vi "ReadCICDPathConfig.vi"(8 "error in (no error)":errorcluster, 11 "Workspace Path":path=path "E:/sw-deps-monitor") -> (0 "error out":errorcluster, 3 "CICD Path Config Out":T1)   [LabVIEW 2023, in "CICD.lvlib"]
uses:
  CICD.lvlib
  Typedefs/CICDPathConfigs.ctl
  <vilib>/Utility/config.llb/NI_LVConfig.lvlib
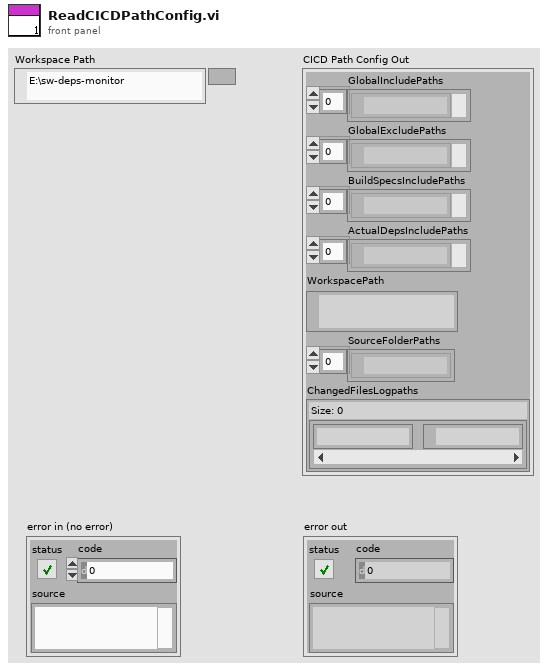
[diagram p1: front panel]
types:
  T1 = typedef "CICD.lvlib/CICDPathConfigs.ctl" = cluster{"GlobalIncludePaths":path[], "GlobalExcludePaths":path[], "BuildSpecsIncludePaths":path[], "ActualDepsIncludePaths":path[], "WorkspacePath":path, "SourceFolderPaths":path[], "ChangedFilesLogpaths":map{string, path}}
  T2 = typedef "NI_LVConfig.lvlib/Config Data RefNum.ctl" = refnum<k1>
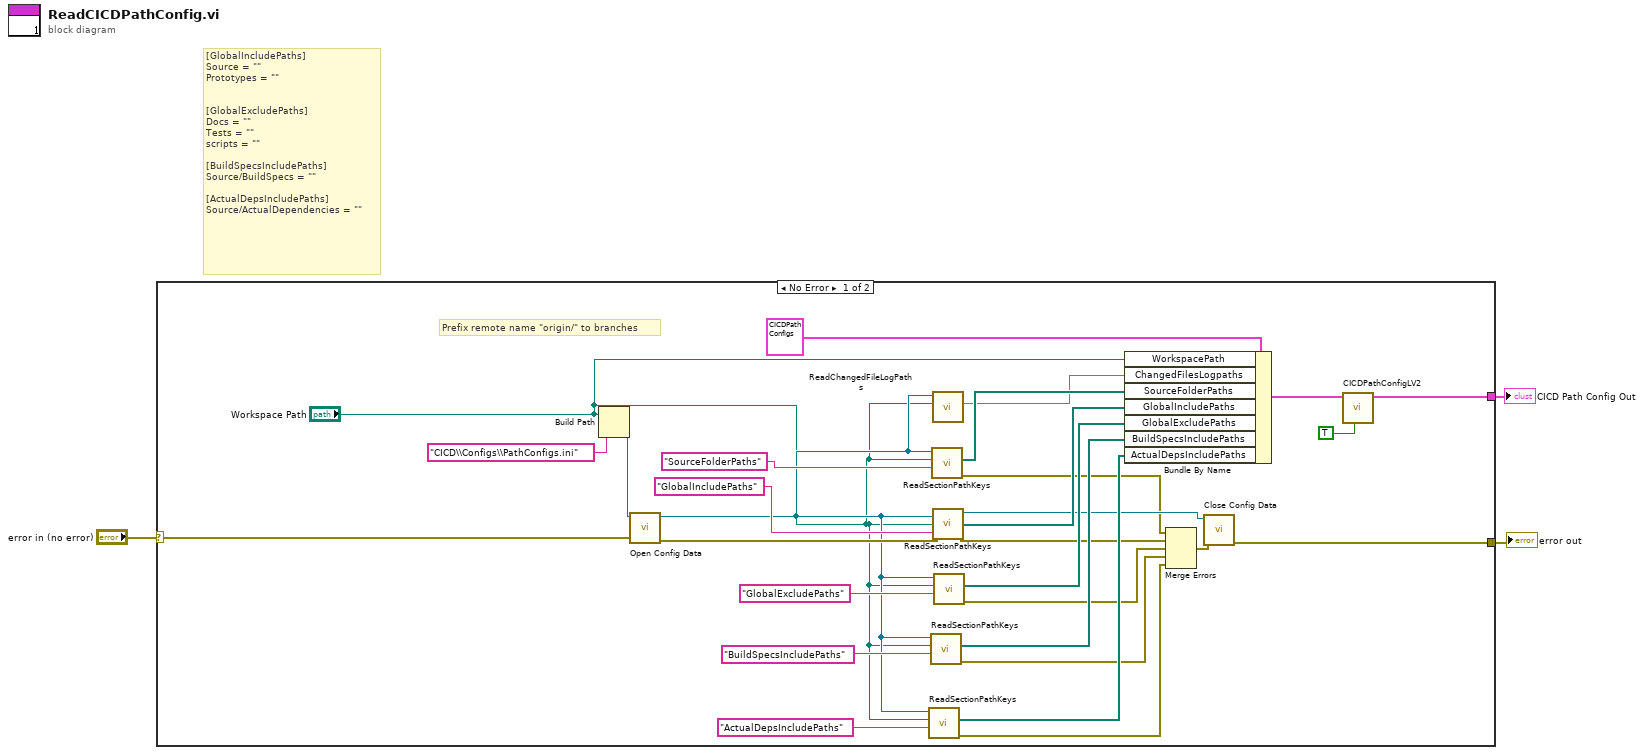
[diagram p0: block diagram]
diagram:
  # "[GlobalIncludePaths]\nSource = \"\"\nPrototypes = \"\"\n\n\n[GlobalExcludePaths]\nDocs = \"\"\nTests = \"\"\nscripts = \"\"\n\n[BuildSpecsIncludePaths]\nSource/BuildSpecs = \"\"\n\n[ActualDepsIncludePaths]\nSource/ActualDependencies = \"\""
  n1 = case shown="No Error" "error in (no error)" {
    selector: "error in (no error)" -> [w32 w33]
    tunnel: [w13 w33] -> w2
    tunnel: [w10 _] -> w1
    frame No Error {
      # "Prefix remote name \"origin/\" to branches"
      n2 = Build Path(base path="Workspace Path", name or relative path="CICD\\Configs\\PathConfigs.ini" ("CICD Path Config Rel")) -> (appended path=w31:path)
      n3 = call <vilib>:"Open Config Data.vi"("error in (no error)"=w32, "configuration file path"=w31) -> ("error out"=w29:errorcluster, "refnum"=w6:T2)  [unwired: 7 in, 1 out]
      n4 = call "ReadSectionPathKeys.vi"("section"="ActualDepsIncludePaths", "Workspace Path"="Workspace Path", "Refnum in"=w6) -> ("error out"=w16:errorcluster, "Paths"=w20:path[])  [unwired: 6 in, 1 out]
      n5 = call "ReadSectionPathKeys.vi"("section"="BuildSpecsIncludePaths", "Workspace Path"="Workspace Path", "Refnum in"=w6) -> ("error out"=w17:errorcluster, "Paths"=w21:path[])  [unwired: 6 in, 1 out]
      n6 = call "ReadSectionPathKeys.vi"("section"="SourceFolderPaths", "Workspace Path"="Workspace Path", "Refnum in"=w6) -> ("error out"=w8:errorcluster, "Paths"=w7:path[])  [unwired: 6 in, 1 out]
      n7 = call "ReadChangedFileLogPaths.vi"("Workspace Path"="Workspace Path", "Refnum in"=w6) -> ("ChangedFilesLogpaths"=w4:map{string, path})  [unwired: 7 in, 2 out]
      n8 = call "ReadSectionPathKeys.vi"("error in (no error)"=w29, "section"="GlobalIncludePaths", "Workspace Path"="Workspace Path", "Refnum in"=w6) -> ("error out"=w19:errorcluster, "Paths"=w23:path[], "refnum out"=w14:T2)  [unwired: 5 in]
      n9 = call "ReadSectionPathKeys.vi"("section"="GlobalExcludePaths", "Workspace Path"="Workspace Path", "Refnum in"=w6) -> ("error out"=w18:errorcluster, "Paths"=w22:path[])  [unwired: 6 in, 1 out]
      n10 = Bundle By Name(cluster=T1 {"GlobalIncludePaths"=[], "GlobalExcludePaths"=[], "BuildSpecsIncludePaths"=[], "ActualDepsIncludePaths"=[], "WorkspacePath"=path "", "SourceFolderPaths"=[], "ChangedFilesLogpaths"={}}, "WorkspacePath"="Workspace Path", "ChangedFilesLogpaths"=w4, "SourceFolderPaths"=w7, "GlobalIncludePaths"=w23, "GlobalExcludePaths"=w22, "BuildSpecsIncludePaths"=w21, "ActualDepsIncludePaths"=w20) -> (w11:T1)
      n11 = Merge Errors(w8, w19, w18, w17, w16) -> (w15:errorcluster)
      n12 = call <vilib>:"Close Config Data.vi"("error in (no error)"=w15, "refnum"=w14) -> ("error out"=w13:errorcluster)  [unwired: 8 in, 1 out]
      n13 = call "CICDPathConfigLV2.vi"("Set? (F)"=TRUE, "CICD Path Config In"=w11) -> ("CICD Path Config Out"=w10:T1)  [unwired: 9 in]
    }
    frame Error {
    }
  }
  "error out" <- w2
  "CICD Path Config Out" <- w1
